vi "Get_Number_Problem_Points_in_Track-1.vi"(1 "[IN] Dot Statuses in Track":i16[](array[numeric])) -> (0 "[OUT] Number of Prob-\nlem Points in Track":i16)   [LabVIEW 2013]
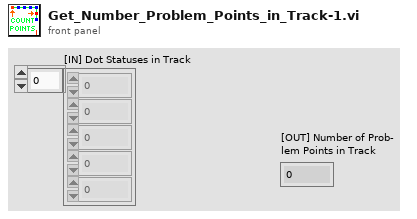
[diagram p1: front panel]
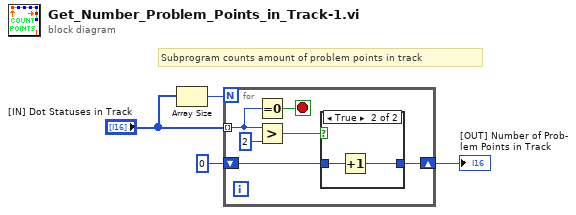
[diagram p0: block diagram]
diagram:
  # "Subprogram counts amount of problem points in track"
  n1 = Array Size(array="[IN] Dot Statuses in Track") -> (size(s)=w4:i32)
  n2 = for {
    N: w4 -> [_]
    shift-right: [w5] -> w1
    shift-left: i16 0 -> [w9]
    tunnel: "[IN] Dot Statuses in Track" -> [w8] mode=indexing
    stop <- w6 stop-if-true
    n3 = Equal To 0?(x=w8) -> (x = 0?=w6:bool)
    n4 = Greater?(x=w8, y=i16 2) -> (0:w7:bool)
    n5 = case shown="True" w7 {
      tunnel: w9 -> [w11 w13]
      tunnel: [w11 w12] -> w5
      frame False {
      }
      frame True {
        n6 = Increment(x=w13) -> (x+1=w12:i16)
      }
    }
  }
  "[OUT] Number of Prob-\nlem Points in Track" <- w1
